vi "Pockels Cal-Cal listbox selector remap.vi"(7 "Function":T1(ring), 8 "error in (no error)":errorcluster, 9 "Filtered Array in":string[](array[string]), 11 "ListBox in":refnum<vi>) -> (0 "error out":errorcluster, 1 "index of element":i32, 3 "ListBox out":refnum<vi>)   [LabVIEW 2017]
uses:
  Globals/gl_Calibration globals.vi
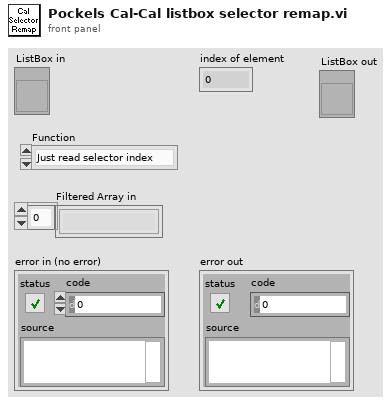
[diagram p1: front panel]
types:
  T1 = enum16{"Just read selector index", "remap to selected cal", "map to active cal"}
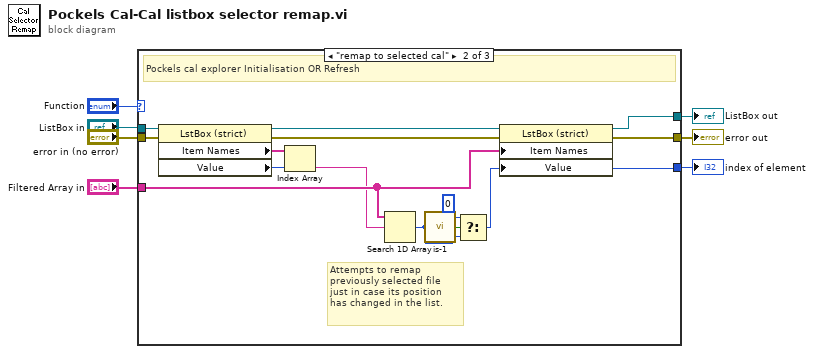
[diagram p0: block diagram]
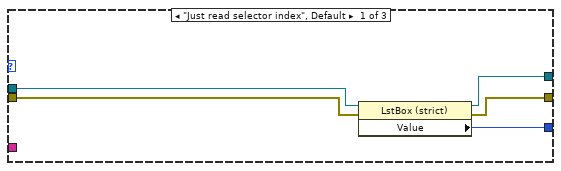
[diagram p2: hidden frame]
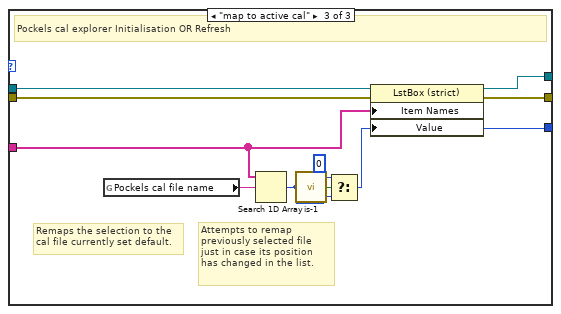
[diagram p3: hidden frame]
diagram:
  n1 = case shown="\"remap to selected cal\"" "Function" {
    tunnel: [w12 w15 w29] -> w3
    tunnel: "Filtered Array in" -> [_ w19 w33]
    tunnel: "ListBox in" -> [w11 w25 w34]
    tunnel: [w10 w26 w36] -> w6
    tunnel: "error in (no error)" -> [w9 w24 w35]
    tunnel: [w8 w13 w27] -> w1
    frame "Just read selector index", Default {
      n2 = property on="Property Node" class="LstBox (strict)"(reference=w11, error in=w9) -> (reference out=w8:refnum<vi>, error out=w10:errorcluster, "Value"=w12:i32)
    }
    frame "remap to selected cal" {
      # "Attempts to remap previously selected file just in case its position has changed in the list."
      # "Pockels cal explorer Initialisation OR Refresh"
      n3 = property on="Property Node" class="LstBox (strict)"(reference=w25, error in=w24) -> (reference out=w22:refnum<vi>, error out=w23:errorcluster, "Item Names"=w21:string[], "Value"=w20:i32)
      n4 = Index Array(array=w21, index=w20) -> (element=w14:string)
      n5 = Search 1D Array(1D array=w19, element=w14) -> (index of element=w16:i32)  [unwired: 1 in]
      n6 = call "is-1.vi"("Value"=w16) -> ("is -1?"=w18:bool)  [unwired: 4 in]
      n7 = Select(t=0 ("Listbox"), s=w18, f=w16) -> (s? t:f=w15:i32)
      n8 = property on="Property Node" class="LstBox (strict)"(reference=w22, error in=w23, "Item Names"=w19, "Value"=w15) -> (reference out=w13:refnum<vi>, error out=w26:errorcluster)
    }
    frame "map to active cal" {
      # "Remaps the selection to the\ncal file currently set default."
      # "Attempts to remap previously selected file just in case its position has changed in the list."
      # "Pockels cal explorer Initialisation OR Refresh"
      n9 = global read "gl_Calibration globals.vi" "Pockels cal file name"() -> (w28:string)
      n10 = Search 1D Array(1D array=w33, element=w28) -> (index of element=w30:i32)  [unwired: 1 in]
      n11 = call "is-1.vi"("Value"=w30) -> ("is -1?"=w32:bool)  [unwired: 4 in]
      n12 = Select(t=0 ("Listbox"), s=w32, f=w30) -> (s? t:f=w29:i32)
      n13 = property on="Property Node" class="LstBox (strict)"(reference=w34, error in=w35, "Item Names"=w33, "Value"=w29) -> (reference out=w27:refnum<vi>, error out=w36:errorcluster)
    }
  }
  "error out" <- w6
  "index of element" <- w3
  "ListBox out" <- w1
